vi "ag33xxx - Display.vi"(6 "Display Text":string, 8 "error in (no error)":errorcluster, 9 "Text (F: off)":bool, 10 "Display (T: On)":bool=TRUE, 11 "VISA session":refnum<visa-resource-name>) -> (0 "error out":errorcluster, 3 "dup VISA session":refnum<visa-resource-name>)   [LabVIEW 2014, in "AFG3352X.lvlib"]
doc: "Turns the front-panel display on or off. Allows the user to write a message on the front-panel display.\n\nThis is an adapted VI that should, in principe, be part of the instrument driver. However, I do not like to patch the original driver. This this VI has been added to the library of the CS class."
uses:
  AFG3352X.lvlib
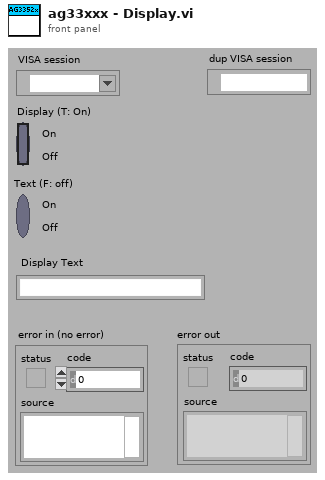
[diagram p1: front panel]
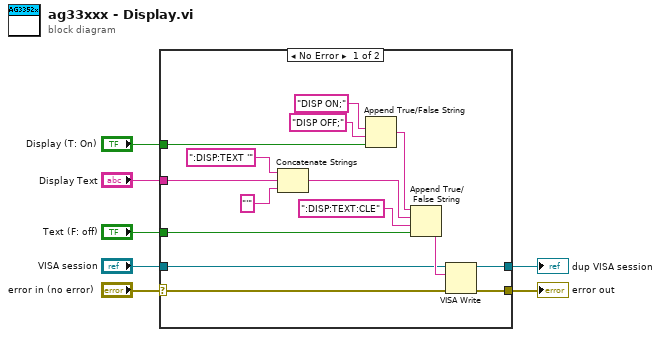
[diagram p0: block diagram]
diagram:
  n1 = case shown="No Error" "error in (no error)" {
    selector: "error in (no error)" -> [w8 w23]
    tunnel: "Display Text" -> [w20 _]
    tunnel: "Display (T: On)" -> [w17 _]
    tunnel: "Text (F: off)" -> [w16 _]
    tunnel: [w14 w23] -> w4
    tunnel: [w12 w24] -> w3
    tunnel: "VISA session" -> [w11 w24]
    frame No Error {
      n2 = Concatenate Strings(":DISP:TEXT '", w20, "'") -> (w19:string)
      n3 = Append True/False String(1:w17, 2:"DISP OFF;", 3:"DISP ON;") -> (0:w18:string)  [unwired: 1 in]
      n4 = Append True/False String(1:w16, 2:":DISP:TEXT:CLE", 3:w19, 4:w18) -> (0:w13:string)
      n5 = VISA Write(VISA resource name=w11, write buffer=w13, error in (no error)=w8) -> (VISA resource name out=w12:refnum<visa-resource-name>, error out=w14:errorcluster)  [unwired: 1 out]
    }
    frame Error {
    }
  }
  "error out" <- w4
  "dup VISA session" <- w3
